vi "FSM Load Pipette.vi"(0 "Dialog Indicator":refnum<vi>, 2 "Pressure Controls":T1, 4 "Reset":refnum<vi>, 5 "error in (no error)":errorcluster, 7 "Disengage Target":refnum<vi>, 9 "Pressure Levels [KPa]":refnum<vi>) -> (19 "error out":errorcluster)   [LabVIEW 2012, in "Autopatcher Daemon.lvlib"]
uses:
  Autopatcher Daemon.lvlib
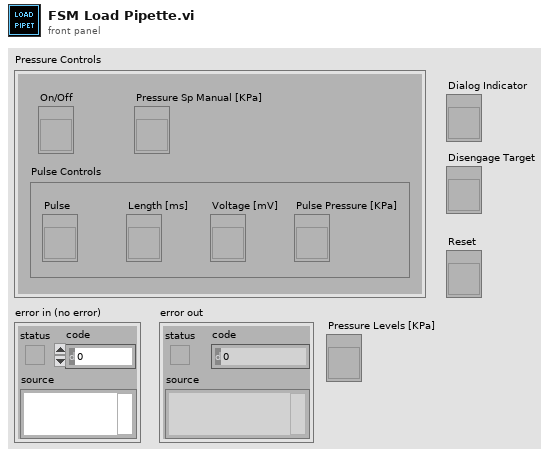
[diagram p1: front panel]
types:
  T1 = cluster{"On/Off":refnum<vi>, "Pulse Controls":cluster{"Pulse":refnum<vi>, "Length [ms]":refnum<vi>, "Voltage [mV]":refnum<vi>, "Pulse Pressure [KPa]":refnum<vi>}, "Pressure Sp Manual [KPa]":refnum<vi>}
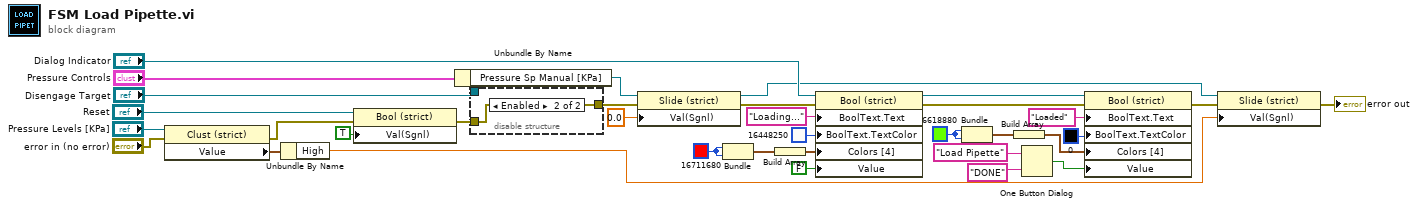
[diagram p0: block diagram]
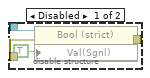
[diagram p2: hidden frame]
diagram:
  w14 = u32 6618880
  w16 = u32 16711680
  n1 = property class="Clust (strict)"(reference="Pressure Levels [KPa]", error in="error in (no error)") -> (error out=w5:errorcluster, "Value"=w6:cluster{"High":dbl, "Low":dbl})  [unwired: 1 out]
  n2 = Unbundle By Name(w6) -> ("High"=w1:dbl)
  n3 = property class="Bool (strict)"(reference="Reset", error in=w5, "Val(Sgnl)"=TRUE ("Value (Signaling)")) -> (error out=w9:errorcluster)  [unwired: 1 out]
  n4 = Unbundle By Name("Pressure Controls") -> ("Pressure Sp Manual [KPa]"=w3:refnum<vi>)
  n5 = disable-structure shown="Enabled" {
    disable-tunnel: "Disengage Target" -> [w38 _]
    disable-tunnel: w9 -> [w36 w39]
    disable-tunnel: [w35 w39] -> w2
    frame Disabled {
      n6 = property class="Bool (strict)"(reference=w38, error in=w36, "Val(Sgnl)"=TRUE ("Value (Signaling)")) -> (error out=w35:errorcluster)  [unwired: 1 out]
    }
    frame Enabled {
    }
  }
  n7 = property class="Slide (strict)"(reference=w3, error in=w2, "Val(Sgnl)"=0.0 ("Value")) -> (reference out=w19:refnum<vi>, error out=w21:errorcluster)
  n8 = Bundle(w16, w16) -> (w17:cluster{u32, u32})  [unwired: 1 in]
  n9 = Build Array(w17) -> (w15:cluster{u32, u32}[])
  n10 = property class="Bool (strict)"(reference="Dialog Indicator", error in=w21, "BoolText.Text"="Loading..." ("Boolean Text.Text"), "BoolText.TextColor"=u32 16448250, "Colors [4]"=w15, "Value"=FALSE) -> (reference out=w23:refnum<vi>, error out=w24:errorcluster)
  n11 = Bundle(w14, w14) -> (w13:cluster{u32, u32})  [unwired: 1 in]
  n12 = Build Array(w13) -> (w12:cluster{u32, u32}[])
  n13 = One Button Dialog(message="Load Pipette", button name ("OK")="DONE") -> (true=w22:bool)
  n14 = property class="Bool (strict)"(reference=w23, error in=w24, "BoolText.Text"="Loaded" ("Boolean Text.Text"), "BoolText.TextColor"=u32 0, "Colors [4]"=w12, "Value"=w22) -> (error out=w20:errorcluster)  [unwired: 1 out]
  n15 = property class="Slide (strict)"(reference=w19, error in=w20, "Val(Sgnl)"=w1) -> (error out=→"error out":errorcluster)  [unwired: 1 out]
